vi "run.vi"(8 "error in (no error)":errorcluster, 11 "DL090409StageScaffold in":refnum<class "StageDL090409Scaffold.lvclass">) -> (0 "error out":errorcluster, 3 "DL090409StageScaffold out":refnum<class "StageDL090409Scaffold.lvclass">)   [LabVIEW 2010, in "StageDL090409Scaffold.lvclass"]
uses:
  StageDL090409Scaffold.lvclass
  main/labview_source/controls/undock_button.ctl
  internal_trigger_enum.ctl
  state_enum.ctl
  common/classes/SpaceVector/SpaceVector/SpaceVector.lvclass
  StageDL090409Scaffold.lvclass/StageDL090409Scaffold.ctl
  common/enumerations/top-level_component_type_enum.ctl
  GenericStage/GenericStage/trigger_enum.ctl
  GenericStage/GenericStage/translation_mode_enum.ctl
  stored_data_cluster.ctl
  common/classes/Image/Image/Image.lvclass
  Display/GenericDisplay/GenericDisplay/GenericDisplay.lvclass
  common/classes/GenericToplevelComponent/GenericToplevelComponent/trigger_type_enum.ctl
  GenericStage/GenericStage/GenericStage.lvclass
  common/classes/GenericToplevelComponent/GenericToplevelComponent/GenericToplevelComponent.lvclass
  common/classes/ErrorController/ErrorController/class_data.vi
  common/classes/ErrorController/ErrorController/ErrorController.lvclass
panel:
  in  "button:undock":T1
  in  "Tab Control":enum32{"User", "Debug", "About"}(tab)
  out "current x":dbl[unit] caption="x"
  out "current y":dbl[unit] caption="y"
  out "current z":dbl[unit] caption="z"
  in  "setOriginButton":bool
  in  "step x":dbl[unit] caption="x"
  in  "step y":dbl[unit] caption="y"
  in  "step z":dbl[unit] caption="z"
  in  "stepButton":bool
  in  "returnToOriginButton":bool
  in  "Stored positions":i32(listbox)
  in  "Description":string
  in  "store button":bool
  out "position image":T2(plugin-control)
  in  "go to stored button":bool
  in  "remove stored item":bool
  out "finished?":bool
  out "last trigger":T3=enum."initialise"
  out "state":T4
  out "statemachine loop counter":i32
  out "event loop error":errorcluster
  out "statemachine error":errorcluster
  out "event loop counter":i32
  # "Move"
  # "Current position"
  # "StageDL090409Scaffold (or child class)\n\nimplemented by: Dominik Langer, University of Zurich\nmodified by: Marcel van 't Hoff, University of Zurich"
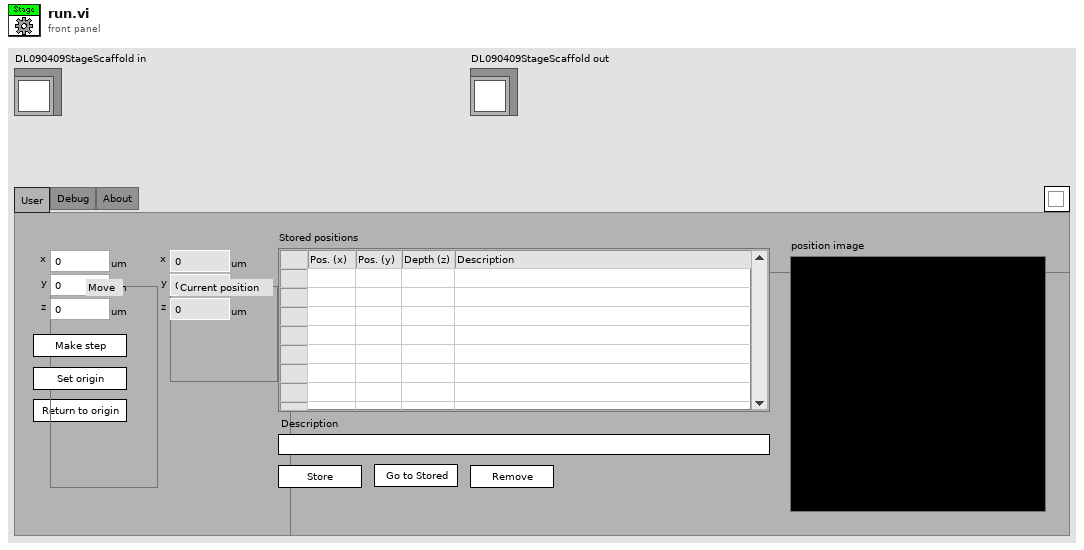
[diagram p1: front panel]
types:
  T1 = typedef "undock_button.ctl" = bool
  T2 = typedef "IMAQ Image.ctl" = refnum<image>
  T3 = typedef "StageDL090409Scaffold.lvclass/internal_trigger_enum.ctl" = enum16{"NULL", "initialise", "terminate", "move", "update position", "set origin", "return to origin", "attach observer", "detach observer", "go to stored"}
  T4 = typedef "StageDL090409Scaffold.lvclass/state_enum.ctl" = enum16{"idle", "moving"}
  T5 = typedef "top-level_component_type_enum.ctl" = enum16{"undefined", "ImagingMode", "ScanHead", "DAQ", "ImageAssembler", "Display", "DataCollection", "Analyser", "Stimulator", "ExperimentController", "Instrument", "Stage"}
  T6 = typedef "GenericStage.lvclass/trigger_enum.ctl" = enum16{"NULL", "move", "update position", "set origin", "return to origin"}
  T7 = typedef "GenericStage.lvclass/translation_mode_enum.ctl" = enum16{"DON'T MOVE", "relative", "absolute"}
  T8 = typedef "StageDL090409Scaffold.lvclass/stored_data_cluster.ctl" = cluster{"stored position":refnum<class "SpaceVector.lvclass">, "description":string, "position image":refnum<class "Image.lvclass">}
  T9 = typedef "trigger_type_enum.ctl" = enum8{"external", "internal", "common"}
  T10 = typedef "main_trigger_enum.ctl" = enum16{"NULL", "initialise", "terminate", "start", "stop", "change objective", "change experimentController", "change imagingMode", "save notebook", "started saving", "finished saving", "expCtr ready", "expCtr missing", "imgMd ready", "imgMd missing", "scanHd ready", "scanHd missing", "DAQ ready", "DAQ missing", "imgAsm ready", "imgAsm missing", "dataColl ready", "dataColl missing", "display ready", "display missing", "analysr ready", "analysr missing", "instrmnt ready", "instrmnt missing", "stimltr ready", "stimltr missing", "stage ready", "stage missing"}
  T11 = typedef "GenericToplevelComponent.lvclass/common_trigger_enum.ctl" = enum16{"NULL", "initialise", "terminate", "fetch command", "fetch data", "attach observer", "register as observer", "detach observer", "acknowledge", "start", "stop", "sweep started", "sweep finished", "experiment started", "experiment stopped"}
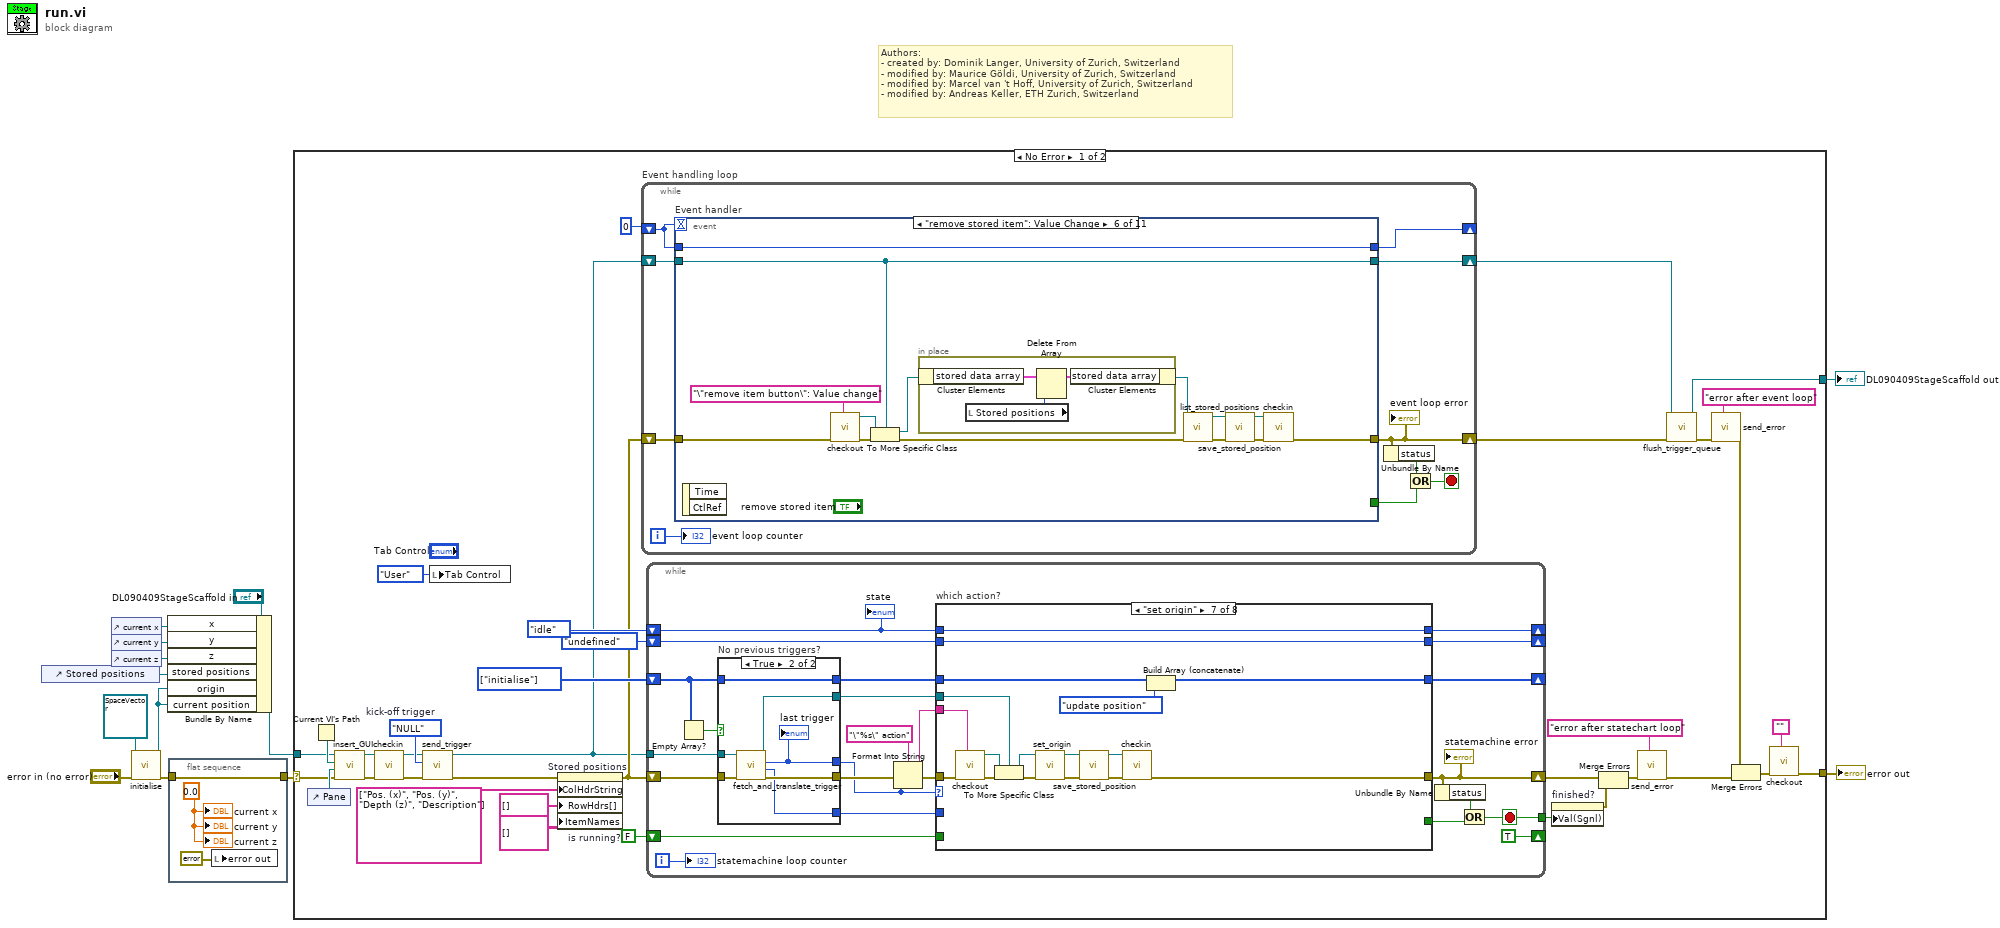
[diagram p0: block diagram]
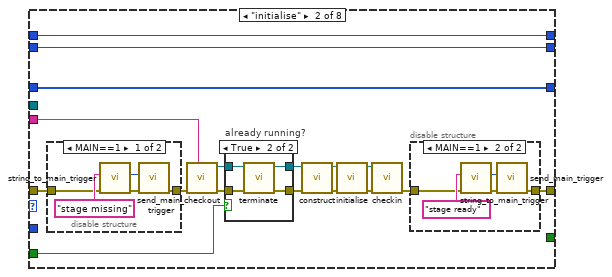
[diagram p3: hidden frame]
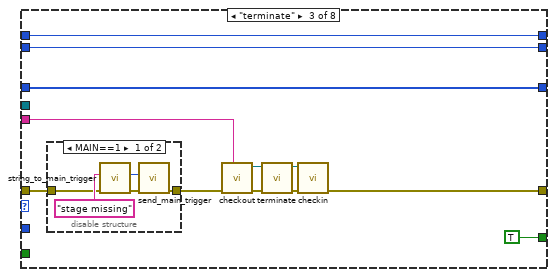
[diagram p7: hidden frame]
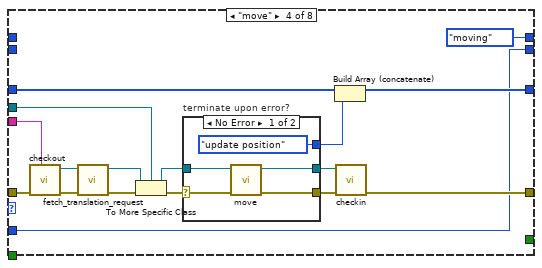
[diagram p9: hidden frame]
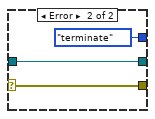
[diagram p10: hidden frame]
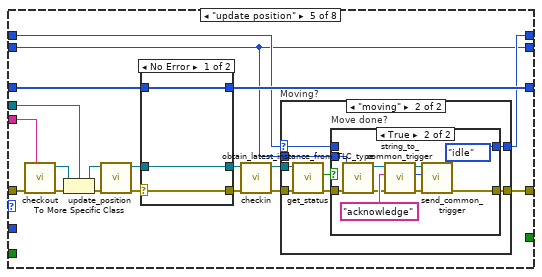
[diagram p11: hidden frame]
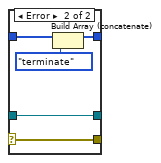
[diagram p14: hidden frame]
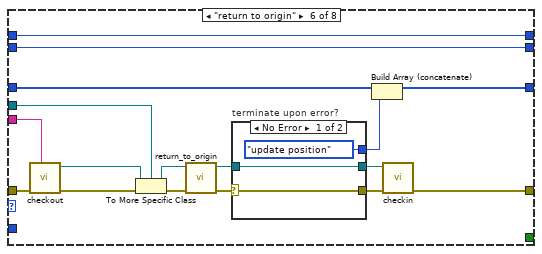
[diagram p15: hidden frame]
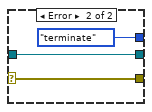
[diagram p16: hidden frame]
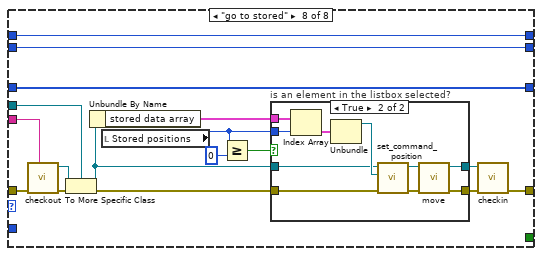
[diagram p17: hidden frame]
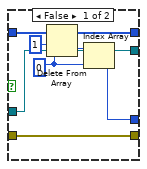
[diagram p19: hidden frame]
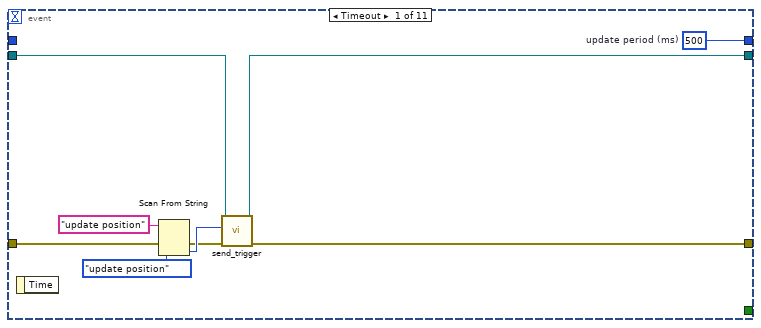
[diagram p20: hidden frame]
diagram:
  # "Authors: \n- created by: Dominik Langer, University of Zurich, Switzerland\n- modified by: Maurice Göldi, University of Zurich, Switzerland\n- modified by: Marcel van 't Hoff, University of Zurich, Switzerland\n- modified by: Andreas Keller, ETH Zurich, Switzerland"
  n1 = control-ref of="Stored positions"() -> (w6:refnum<vi>)
  n2 = control-ref of="current x"() -> (w9:refnum<vi>)
  n3 = control-ref of="current y"() -> (w8:refnum<vi>)
  n4 = control-ref of="current z"() -> (w7:refnum<vi>)
  n5 = call "initialise.vi"("error in (no error)"="error in (no error)", "SpaceVector in"=refnum<class "SpaceVector.lvclass"> refnum ("current position")) -> ("error out"=w2:errorcluster, "SpaceVector out"=w4:refnum<class "SpaceVector.lvclass">)  [unwired: 3 in, 5 out]
  n6 = Bundle By Name(cluster="DL090409StageScaffold in", "x"=w9, "y"=w8, "z"=w7, "stored positions"=w6, "origin"=w4, "current position"=w4) -> (w10:refnum<class "StageDL090409Scaffold.lvclass">)
  n7 = flat-sequence {
    tunnel: w2 -> [w15]
    tunnel: [w15] -> w1
    frame #0 {
      w16 = dbl[unit] 0.0 ("current x")
      n8 = local write "error out"(errorcluster {"status"=FALSE, "code"=0, "source"=""} ("error in (no error)")) -> ()
      "current x" <- w16
      "current y" <- w16
      "current z" <- w16
    }
  }
  n9 = case shown="No Error" w1 {
    selector: w1 -> [w44 w458]
    tunnel: [w50 w458] -> w13
    tunnel: [w31 w457] -> w12
    tunnel: w10 -> [w47 w457]
    frame No Error {
      w29 = FALSE  # is running?
      w30 = T3[] [enum."initialise"] items=["NULL", "initialise", "terminate", "move", "update position", "set origin", "return to origin", "attach observer", "detach observer", "go to stored"]
      w40 = trigger_enum."NULL"  # kick-off trigger
      n10 = control-ref of="Pane"() -> (w46:refnum<vi>)
      n11 = Current VI's Path() -> (path=w48:path)
      n12 = call-dynamic "insert_GUI.vi"("error in (no error)"=w44, "Pane"=w46, "VI path"=w48, "GenericComponent in"=w47) -> ("error out"=w22:errorcluster, "GenericComponent out"=w21:refnum<class "StageDL090409Scaffold.lvclass">)  [unwired: 6 in]
      n13 = call-dynamic "checkin.vi"("error in (no error)"=w22, "GenericStage in"=w21) -> ("error out"=w38:errorcluster, "GenericStage out"=w37:refnum<class "StageDL090409Scaffold.lvclass">)  [unwired: 8 in]
      n14 = call-dynamic "send_trigger.vi"("error in (no error)"=w38, "trigger"=w40, "GenericStage in"=w37) -> ("error out"=w41:errorcluster, "GenericStage out"=w19:refnum<class "StageDL090409Scaffold.lvclass">)  [unwired: 7 in]
      n15 = local write "Tab Control"(enum32{"User", "Debug", "About"}."User" ("Tab Control")) -> ()
      n16 = property on="Stored positions" class="MCListbox (strict)"(error in=w41, "ColHdrString"=string[] ["Pos. (x)", "Pos. (y)", "Depth (z)", "Description"] ("Row Header Strings[]"), "RowHdrs[]"=string[] [] ("Row Header Strings[]"), "ItemNames"=string[][] [] ("Item Names")) -> (error out=w20:errorcluster)  [unwired: 1 in, 1 out]
      n17 = while "Event handling loop" {
        shift-right: [w300] -> _
        shift-left: 0 -> [w301]
        shift-right: [w296] -> w33
        shift-left: w20 -> [w299]
        shift-right: [w297] -> w34
        shift-left: w19 -> [w298]
        i -> [w292]
        stop <- w293 stop-if-true
        n18 = event "Event handler" shown="[5] \"remove stored item\": Value Change" {
          selector: _ -> [_ _ _ _ _ _ _ _ _ _ _]
          dyn-events: _ -> [_ _ _ _ _ _ _ _ _ _ _]
          timeout: w301 -> [_ _ _ _ _ _ _ _ _ _ _]
          tunnel: w301 -> [_ w319 w331 w340 w372 w399 w413 w428 w435 w452 w456]
          tunnel: [w310 w319 w331 w340 w372 w399 w413 w428 w435 w452 w456] -> w300
          tunnel: w299 -> [w303 w317 w330 w334 w371 w394 w412 w421 w434 w451 w455]
          tunnel: [w307 w311 w324 w337 w347 w393 w409 w415 w433 w447 w455] -> w296
          tunnel: [_ _ _ _ _ _ _ _ _ _ TRUE] -> w294
          tunnel: w298 -> [w309 w318 w323 w339 w368 w398 w408 w417 w432 w444 w453]
          tunnel: [w308 w312 w321 w338 w368 w398 w407 w417 w431 w443 w453] -> w297
          event Timeout {
            w310 = 500  # update period (ms)
            n19 = event-data() -> ()  [unwired: 2 out]
            n20 = Scan From String(input string="update position", error in=w303, default 1=trigger_enum."update position" ("trigger")) -> (error out=w302:errorcluster, output 1=w304:T6)  [unwired: 2 in, 2 out]
            n21 = call-dynamic "send_trigger.vi"("error in (no error)"=w302, "trigger"=w304, "GenericStage in"=w309) -> ("error out"=w307:errorcluster, "GenericStage out"=w308:refnum<class "StageDL090409Scaffold.lvclass">)  [unwired: 7 in]
          }
          event "setOriginButton": Value Change {
            n22 = event-data() -> ()  [unwired: 3 out]
            n23 = Scan From String(input string="set origin", error in=w317, default 1=trigger_enum."set origin" ("trigger")) -> (error out=w316:errorcluster, output 1=w313:T6)  [unwired: 2 in, 2 out]
            n24 = call-dynamic "send_trigger.vi"("error in (no error)"=w316, "trigger"=w313, "GenericStage in"=w318) -> ("error out"=w311:errorcluster, "GenericStage out"=w312:refnum<class "StageDL090409Scaffold.lvclass">)  [unwired: 7 in]
          }
          event "stepButton": Value Change {
            n25 = event-data() -> ()  [unwired: 3 out]
            n26 = call "initialise.vi"("z"="step z", "error in (no error)"=w330, "y"="step y", "x"="step x", "SpaceVector in"=refnum<class "SpaceVector.lvclass"> refnum ("current position")) -> ("error out"=w325:errorcluster, "SpaceVector out"=w326:refnum<class "SpaceVector.lvclass">)  [unwired: 5 in]
            n27 = call-dynamic "send_translation_request.vi"("error in (no error)"=w325, "translation mode"=translation_mode_enum."relative", "translation vector"=w326, "GenericStage in"=w323) -> ("error out"=w324:errorcluster, "GenericStage out"=w321:refnum<class "StageDL090409Scaffold.lvclass">)  [unwired: 6 in]
          }
          event "returnToOriginButton": Value Change {
            n28 = event-data() -> ()  [unwired: 3 out]
            n29 = Scan From String(input string="return to origin", error in=w334, default 1=trigger_enum."return to origin" ("trigger")) -> (error out=w333:errorcluster, output 1=w332:T6)  [unwired: 2 in, 2 out]
            n30 = call-dynamic "send_trigger.vi"("error in (no error)"=w333, "trigger"=w332, "GenericStage in"=w339) -> ("error out"=w337:errorcluster, "GenericStage out"=w338:refnum<class "StageDL090409Scaffold.lvclass">)  [unwired: 7 in]
          }
          event "store button": Value Change {
            n31 = event-data() -> ()  [unwired: 3 out]
            n32 = call "checkout.vi"("locked by?"="\"store button\": Value change", "error in (no error)"=w371) -> ("error out"=w370:errorcluster, "GenericStage out"=w369:refnum<class "GenericStage.lvclass">)  [unwired: 8 in]
            n33 = To More Specific Class(target class=w368, reference=w369, error in=w370) -> (specific class reference=w355:refnum<class "StageDL090409Scaffold.lvclass">, error out=w363:errorcluster)
            n34 = Unbundle By Name(w355) -> ("stored data array"=w357:T8[], "current position"=w360:refnum<class "SpaceVector.lvclass">)
            n35 = call "create.vi"("error in (no error)"=w363) -> ("error out"=w362:errorcluster, "Image out"=w361:refnum<class "Image.lvclass">)  [unwired: 9 in]
            n36 = disable-structure shown="DISPLAY==1" {
              disable-tunnel: w362 -> [w375 w378]
              disable-tunnel: [w374 w378] -> w352
              disable-tunnel: [w373 _] -> w350
              frame condition #0 (active) {
                n37 = call "obtain_latest_instance.vi"("error in (no error)"=w375) -> ("error out"=w377:errorcluster, "GenericDisplay out"=w376:refnum<class "GenericDisplay.lvclass">)  [unwired: 9 in]
                n38 = call-dynamic "get_current_RGB_image.vi"("error in (no error)"=w377, "GenericDisplay in"=w376) -> ("error out"=w374:errorcluster, "RGB image"=w373:refnum<class "Image.lvclass">)  [unwired: 7 in, 1 out]
              }
              frame condition #1 {
              }
            }
            n39 = call-dynamic "is_empty.vi"("error in (no error)"=w352, "Image in"=w350) -> ("error out"=w351:errorcluster, "emtpy?"=w348:bool, "Image out"=w349:refnum<class "Image.lvclass">)  [unwired: 7 in]
            n40 = case shown="False" w348 {
              tunnel: [w383 w385] -> w367
              tunnel: [w382 w384] -> w365
              tunnel: w361 -> [w381 w384]
              tunnel: w351 -> [w380 w385]
              tunnel: w349 -> [w379 _]
              frame False {
                n41 = call "copy.vi"("error in (no error)"=w380, "image to copy (source)"=w379, "Image in (target)"=w381) -> ("error out"=w383:errorcluster, "Image out"=w382:refnum<class "Image.lvclass">)  [unwired: 7 in]
              }
              frame True {
              }
            }
            n42 = call-dynamic "get_IMAQ_ref.vi"("error in (no error)"=w367, "Image.lvclass in"=w365) -> ("error out"=w346:errorcluster, "Image"=→"position image":T2, "Image.lvclass out"=w358:refnum<class "Image.lvclass">)  [unwired: 5 in, 2 out]
            n43 = Bundle(cluster=T8 {"stored position"=refnum, "description"="", "position image"=refnum} ("stored data"), "stored position"=w360, "description"="Description", "position image"=w358) -> (w356:T8)
            n44 = Build Array (concatenate)(w357, w356) -> (w353:T8[])
            n45 = Bundle By Name(cluster=w355, "stored data array"=w353) -> (w345:refnum<class "StageDL090409Scaffold.lvclass">)
            n46 = call-dynamic "list_stored_positions.vi"("error in (no error)"=w346, "StageDL090409Scaffold in"=w345) -> ("error out"=w344:errorcluster, "StageDL090409Scaffold out"=w343:refnum<class "StageDL090409Scaffold.lvclass">)  [unwired: 8 in]
            n47 = call-dynamic "save_stored_position.vi"("error in (no error)"=w344, "StageDL090409Scaffold in"=w343) -> ("error out"=w341:errorcluster, "StageDL090409Scaffold out"=w342:refnum<class "StageDL090409Scaffold.lvclass">)  [unwired: 8 in]
            n48 = call-dynamic "checkin.vi"("error in (no error)"=w341, "GenericStage in"=w342) -> ("error out"=w347:errorcluster)  [unwired: 8 in, 1 out]
          }
          event "remove stored item": Value Change {
            n49 = event-data() -> ()  [unwired: 3 out]
            n50 = call "checkout.vi"("locked by?"="\"remove item button\": Value change", "error in (no error)"=w394) -> ("error out"=w397:errorcluster, "GenericStage out"=w395:refnum<class "GenericStage.lvclass">)  [unwired: 8 in]
            n51 = To More Specific Class(target class=w398, reference=w395, error in=w397) -> (specific class reference=w391:refnum<class "StageDL090409Scaffold.lvclass">, error out=w392:errorcluster)
            n52 = in-place {
              n53 = in-place-cluster #1(w391) -> ("stored data array"=w401:T8[])
              n54 = local read "Stored positions"() -> (w402:i32)
              n55 = Delete From Array(array=w401, index=w402) -> (array with subset deleted=w400:T8[])  [unwired: 1 in, 1 out]
              n56 = in-place-cluster #1("stored data array"=w400) -> (w390:refnum<class "StageDL090409Scaffold.lvclass">)
            }
            n57 = call-dynamic "list_stored_positions.vi"("error in (no error)"=w392, "StageDL090409Scaffold in"=w390) -> ("error out"=w389:errorcluster, "StageDL090409Scaffold out"=w387:refnum<class "StageDL090409Scaffold.lvclass">)  [unwired: 8 in]
            n58 = call-dynamic "save_stored_position.vi"("error in (no error)"=w389, "StageDL090409Scaffold in"=w387) -> ("error out"=w388:errorcluster, "StageDL090409Scaffold out"=w386:refnum<class "StageDL090409Scaffold.lvclass">)  [unwired: 8 in]
            n59 = call-dynamic "checkin.vi"("error in (no error)"=w388, "GenericStage in"=w386) -> ("error out"=w393:errorcluster)  [unwired: 8 in, 1 out]
          }
          event "go to stored button": Value Change {
            n60 = event-data() -> ()  [unwired: 2 out]
            n61 = Scan From String(input string="go to stored", error in=w412, default 1=internal_trigger_enum."update position" ("internal trigger")) -> (error out=w410:errorcluster, output 1=w406:T3)  [unwired: 2 in, 2 out]
            n62 = To Variant(anything=w406) -> (Variant=w405:variant)
            n63 = call-dynamic "send_generic_trigger.vi"("error in (no error)"=w410, "trigger type"=trigger_type_enum."internal", "trigger variant"=w405, "GenericToplevelComponent in"=w408) -> ("error out"=w409:errorcluster, "GenericToplevelComponent out"=w407:refnum<class "StageDL090409Scaffold.lvclass">)  [unwired: 4 in, 2 out]
          }
          event "Stored positions": Mouse Up {
            n64 = event-data() -> ()  [unwired: 2 out]
            n65 = call "checkout.vi"("locked by?"="stored positions: Mouse Down", "error in (no error)"=w421) -> ("error out"=w422:errorcluster, "GenericStage out"=w418:refnum<class "GenericStage.lvclass">)  [unwired: 8 in]
            n66 = To More Specific Class(target class=w417, reference=w418, error in=w422) -> (specific class reference=w414:refnum<class "StageDL090409Scaffold.lvclass">, error out=w420:errorcluster)
            n67 = Unbundle By Name(w414) -> ("stored data array"=w427:T8[])
            n68 = Index Array(array=w427, index="Stored positions") -> (element=w426:T8)
            n69 = Unbundle By Name(w426) -> ("position image"=w425:refnum<class "Image.lvclass">)
            n70 = call-dynamic "get_IMAQ_ref.vi"("error in (no error)"=w420, "Image.lvclass in"=w425) -> ("error out"=w416:errorcluster, "Image"=w424:T2)  [unwired: 5 in, 3 out]
            n71 = local write "position image"(w424) -> ()
            n72 = call-dynamic "checkin.vi"("error in (no error)"=w416, "GenericStage in"=w414) -> ("error out"=w415:errorcluster)  [unwired: 8 in, 1 out]
          }
          event Value Change {
            n73 = event-data() -> ()  [unwired: 2 out]
            n74 = Current VI's Path() -> (path=w429:path)
            n75 = call-dynamic "undock.vi"("error in (no error)"=w434, "undock?"="button:undock", "VI path"=w429, "GenericComponent in"=w432) -> ("error out"=w433:errorcluster, "GenericComponent out"=w431:refnum<class "StageDL090409Scaffold.lvclass">)  [unwired: 6 in]
          }
          event "Stored positions": Edit Cell {
            n76 = event-data() -> ("Coords.Row"=w440:i32, "Coords.Column"=w442:i32, "String"=w441:string)  [unwired: 1 out]
            n77 = call "checkout.vi"("locked by?"="Stored position edited: Value Change", "error in (no error)"=w451) -> ("error out"=w448:errorcluster, "GenericStage out"=w449:refnum<class "GenericStage.lvclass">)  [unwired: 8 in]
            n78 = To More Specific Class(target class=w444, reference=w449, error in=w448) -> (specific class reference=w446:refnum<class "StageDL090409Scaffold.lvclass">, error out=w445:errorcluster)
            n79 = call-dynamic "change_stored_position.vi"("Row"=w440, "String"=w441, "Column"=w442, "error in (no error)"=w445, "specific class reference"=w446, "StageDL090409Scaffold in"=w444) -> ("error out"=w439:errorcluster, "specific class reference out"=w436:refnum<class "StageDL090409Scaffold.lvclass">, "StageDL090409Scaffold out"=w443:refnum<class "StageDL090409Scaffold.lvclass">)  [unwired: 3 in]
            n80 = call-dynamic "save_stored_position.vi"("error in (no error)"=w439, "StageDL090409Scaffold in"=w436) -> ("error out"=w437:errorcluster, "StageDL090409Scaffold out"=w438:refnum<class "StageDL090409Scaffold.lvclass">)  [unwired: 8 in]
            n81 = call-dynamic "checkin.vi"("error in (no error)"=w437, "GenericStage in"=w438) -> ("error out"=w447:errorcluster)  [unwired: 8 in, 1 out]
          }
          event "finished?": Value Change {
            n82 = event-data() -> ()  [unwired: 3 out]
          }
        }
        "event loop error" <- w296
        n83 = Unbundle By Name(w296) -> ("status"=w295:bool)
        n84 = Or(x=w295, y=w294) -> (x .or. y?=w293:bool)
        "event loop counter" <- w292
      }
      n85 = while {
        shift-right: [w61] -> w25
        shift-left: w20 -> [w76]
        shift-right: [w67] -> _
        shift-left: w30 -> [w73]
        shift-right: [TRUE ("is running?")] -> _
        shift-left: w29 -> [w64]
        tunnel: w19 -> [w75]
        tunnel: [w58] -> w28
        shift-right: [w56] -> _
        shift-left: state_enum."idle" ("state") -> [w57]
        shift-right: [w54] -> _
        shift-left: top-level_component_type_enum."undefined" ("sender TLC type") -> [w53]
        i -> [w55]
        stop <- w58 stop-if-true
        n86 = Empty Array?(array=w73) -> (empty?=w74:bool)
        n87 = case "No previous triggers?" shown="True" w74 {
          tunnel: w75 -> [w284 w288]
          tunnel: w76 -> [w282 w290]
          tunnel: [w284 w287] -> w68
          tunnel: [w280 w285] -> w70
          tunnel: [_ w286] -> w62
          tunnel: [w282 w289] -> w71
          tunnel: w73 -> [w283 w291]
          tunnel: [w279 w291] -> w66
          frame False {
            w277 = 0 ("index")
            n88 = Delete From Array(array=w283, length=1, index=w277) -> (deleted portion=w281:T3[], array with subset deleted=w279:T3[])
            n89 = Index Array(array=w281, index=w277) -> (element=w280:T3)
          }
          frame True {
            n90 = call-dynamic "fetch_and_translate_trigger.vi"("error in (no error)"=w290, "StageDL090409Scaffold in"=w288) -> ("error out"=w289:errorcluster, "sender TLC type"=w286:T5, "statechart trigger"=w285:T3, "StageDL090409Scaffold out"=w287:refnum<class "StageDL090409Scaffold.lvclass">)  [unwired: 6 in]
            "last trigger" <- w285
          }
        }
        n91 = Format Into String(format string="\"%s\" action", error in=w71, w70) -> (resulting string=w65:string, error out=w69:errorcluster)  [unwired: 1 in]
        n92 = case "which action?" shown="\"set origin\"" w70 {
          tunnel: [w79 w86 w124 w141 w165 w219 w241 w250] -> w61
          tunnel: w69 -> [w79 w84 w117 w148 w176 w223 w245 w251]
          tunnel: w68 -> [_ _ _ w145 w175 w222 w242 w249]
          tunnel: [w80 w85 w127 w139 w169 w211 w239 w264] -> w67
          tunnel: w66 -> [w80 w85 w127 w140 w170 w210 w240 w264]
          tunnel: w65 -> [_ w91 w121 w149 w177 w224 w237 w248]
          tunnel: w64 -> [_ w92 _ _ _ _ _ _]
          tunnel: w62 -> [_ _ _ w134 _ _ _ _]
          tunnel: [_ _ TRUE _ _ _ _ _] -> w60
          tunnel: [w78 w82 w119 state_enum."moving" ("state") w164 w209 w236 w263] -> w56
          tunnel: w57 -> [w78 w82 w119 _ w161 w209 w236 w263]
          tunnel: [w77 w81 w118 w134 w159 w208 w235 w262] -> w54
          tunnel: w53 -> [w77 w81 w118 _ w159 w208 w235 w262]
          frame "NULL", Default {
          }
          frame "initialise" {
            n93 = disable-structure shown="MAIN==1" {
              disable-tunnel: w84 -> [w99 w103]
              disable-tunnel: [w102 w103] -> w83
              frame condition #0 (active) {
                n94 = call "string_to_main_trigger.vi"("error in (no error)"=w99, "trigger string"="stage missing") -> ("error out"=w100:errorcluster, "main trigger"=w98:T10)  [unwired: 8 in]
                n95 = call "send_main_trigger.vi"("error in (no error)"=w100, "trigger"=w98) -> ("error out"=w102:errorcluster)  [unwired: 9 in]
              }
              frame condition #1 {
              }
            }
            n96 = call "checkout.vi"("locked by?"=w91, "error in (no error)"=w83) -> ("error out"=w93:errorcluster, "GenericStage out"=w90:refnum<class "GenericStage.lvclass">)  [unwired: 8 out]
            n97 = case "already running?" shown="True" w92 {
              tunnel: w93 -> [w110 w114]
              tunnel: w90 -> [w111 w115]
              tunnel: [w110 w113] -> w88
              tunnel: [w111 w112] -> w89
              frame False {
              }
              frame True {
                n98 = call-dynamic "terminate.vi"("error in (no error)"=w114, "GenericPlugin in"=w115) -> ("error out"=w113:errorcluster, "GenericPlugin out"=w112:refnum<class "GenericStage.lvclass">)  [unwired: 8 out]
              }
            }
            n99 = call-dynamic "construct.vi"("error in (no error)"=w88, "GenericPlugin in"=w89) -> ("error out"=w95:errorcluster, "GenericPlugin out"=w94:refnum<class "GenericStage.lvclass">)  [unwired: 2 in, 6 out]
            n100 = call-dynamic "initialise.vi"("error in (no error)"=w95, "GenericPlugin in"=w94) -> ("error out"=w96:errorcluster, "GenericPlugin out"=w97:refnum<class "GenericStage.lvclass">)  [unwired: 8 out]
            n101 = call-dynamic "checkin.vi"("error in (no error)"=w96, "GenericStage in"=w97) -> ("error out"=w87:errorcluster)  [unwired: 8 in, 1 out]
            n102 = disable-structure shown="MAIN==1" {
              disable-tunnel: [w104 w109] -> w86
              disable-tunnel: w87 -> [w104 w107]
              frame condition #0 {
              }
              frame condition #1 (active) {
                n103 = call "string_to_main_trigger.vi"("error in (no error)"=w107, "trigger string"="stage ready") -> ("error out"=w106:errorcluster, "main trigger"=w105:T10)  [unwired: 8 in]
                n104 = call "send_main_trigger.vi"("error in (no error)"=w106, "trigger"=w105) -> ("error out"=w109:errorcluster)  [unwired: 9 in]
              }
            }
          }
          frame "terminate" {
            n105 = disable-structure shown="MAIN==1" {
              disable-tunnel: w117 -> [w129 w133]
              disable-tunnel: [w132 w133] -> w116
              frame condition #0 (active) {
                n106 = call "string_to_main_trigger.vi"("error in (no error)"=w129, "trigger string"="stage missing") -> ("error out"=w130:errorcluster, "main trigger"=w128:T10)  [unwired: 8 in]
                n107 = call "send_main_trigger.vi"("error in (no error)"=w130, "trigger"=w128) -> ("error out"=w132:errorcluster)  [unwired: 9 in]
              }
              frame condition #1 {
              }
            }
            n108 = call "checkout.vi"("locked by?"=w121, "error in (no error)"=w116) -> ("error out"=w125:errorcluster, "GenericStage out"=w123:refnum<class "GenericStage.lvclass">)  [unwired: 8 out]
            n109 = call-dynamic "terminate.vi"("error in (no error)"=w125, "GenericPlugin in"=w123) -> ("error out"=w126:errorcluster, "GenericPlugin out"=w122:refnum<class "GenericStage.lvclass">)  [unwired: 8 out]
            n110 = call-dynamic "checkin.vi"("error in (no error)"=w126, "GenericStage in"=w122) -> ("error out"=w124:errorcluster)  [unwired: 8 in, 1 out]
          }
          frame "move" {
            n111 = call "checkout.vi"("locked by?"=w149, "error in (no error)"=w148) -> ("error out"=w150:errorcluster, "GenericStage out"=w147:refnum<class "GenericStage.lvclass">)  [unwired: 8 out]
            n112 = call-dynamic "fetch_translation_request.vi"("error in (no error)"=w150, "GenericStage in"=w147) -> ("error out"=w146:errorcluster, "GenericStage out"=w144:refnum<class "GenericStage.lvclass">)  [unwired: 8 out]
            n113 = To More Specific Class(target class=w145, reference=w144, error in=w146) -> (specific class reference=w137:refnum<class "StageDL090409Scaffold.lvclass">, error out=w136:errorcluster)
            n114 = case "terminate upon error?" shown="No Error" w136 {
              selector: w136 -> [w154 w158]
              tunnel: w137 -> [w155 w157]
              tunnel: [w153 w157] -> w143
              tunnel: [w152 w158] -> w142
              tunnel: [internal_trigger_enum."update position" ("internal trigger enum") internal_trigger_enum."terminate" ("internal trigger enum")] -> w138
              frame No Error {
                n115 = call-dynamic "move.vi"("error in (no error)"=w154, "DL090409StageScaffold in"=w155) -> ("error out"=w152:errorcluster, "DL090409StageScaffold out"=w153:refnum<class "StageDL090409Scaffold.lvclass">)  [unwired: 8 out]
              }
              frame Error {
              }
            }
            n116 = Build Array (concatenate)(w140, w138) -> (w139:T3[])
            n117 = call-dynamic "checkin.vi"("error in (no error)"=w142, "GenericStage in"=w143) -> ("error out"=w141:errorcluster)  [unwired: 8 in, 1 out]
          }
          frame "update position" {
            n118 = call "checkout.vi"("locked by?"=w177, "error in (no error)"=w176) -> ("error out"=w167:errorcluster, "GenericStage out"=w168:refnum<class "GenericStage.lvclass">)  [unwired: 8 out]
            n119 = To More Specific Class(target class=w175, reference=w168, error in=w167) -> (specific class reference=w174:refnum<class "StageDL090409Scaffold.lvclass">, error out=w173:errorcluster)
            n120 = call-dynamic "update_position.vi"("error in (no error)"=w173, "DL090409StageScaffold in"=w174) -> ("error out"=w171:errorcluster, "DL090409StageScaffold out"=w172:refnum<class "StageDL090409Scaffold.lvclass">)  [unwired: 8 out]
            n121 = case shown="No Error" w171 {
              selector: w171 -> [w200 w207]
              tunnel: w172 -> [w201 w206]
              tunnel: [w201 w206] -> w163
              tunnel: [w200 w207] -> w162
              tunnel: w170 -> [w202 w205]
              tunnel: [w202 w204] -> w169
              frame No Error {
              }
              frame Error {
                n122 = Build Array (concatenate)(w205, internal_trigger_enum."terminate" ("internal trigger enum")) -> (w204:T3[])
              }
            }
            n123 = call-dynamic "checkin.vi"("error in (no error)"=w162, "GenericStage in"=w163) -> ("error out"=w166:errorcluster, "GenericStage out"=w160:refnum<class "StageDL090409Scaffold.lvclass">)  [unwired: 8 in]
            n124 = case "Moving?" shown="\"moving\"" w161 {
              selector: w161 -> [w178 w181]
              tunnel: w166 -> [w179 w185]
              tunnel: [w179 w187] -> w165
              tunnel: [w178 w180] -> w164
              tunnel: w160 -> [_ w186]
              tunnel: w159 -> [_ w183]
              frame "idle", Default {
              }
              frame "moving" {
                n125 = call-dynamic "get_status.vi"("error in (no error)"=w185, "StageDL090409Scaffold in"=w186) -> ("error out"=w184:errorcluster, "is happy?"=w182:bool)  [unwired: 7 in, 1 out]
                n126 = case "Move done?" shown="True" w182 {
                  tunnel: [w188 w199] -> w187
                  tunnel: w184 -> [w188 w198]
                  tunnel: w183 -> [_ w197]
                  tunnel: w181 -> [w189 _]
                  tunnel: [w189 state_enum."idle" ("state")] -> w180
                  frame False {
                  }
                  frame True {
                    n127 = call "obtain_latest_instance_from_TLC_type.vi"("error in (no error)"=w198, "top-level component type"=w197) -> ("error out"=w194:errorcluster, "GenericToplevelComponent.lvclass"=w190:refnum<class "GenericToplevelComponent.lvclass">)  [unwired: 8 in]
                    n128 = call-dynamic "string_to_common_trigger.vi"("error in (no error)"=w194, "trigger string"="acknowledge", "GenericToplevelComponent in"=w190) -> ("error out"=w193:errorcluster, "trigger"=w191:T11, "GenericToplevelComponent out"=w192:refnum<class "GenericToplevelComponent.lvclass">)  [unwired: 6 in]
                    n129 = call-dynamic "send_common_trigger.vi"("error in (no error)"=w193, "trigger"=w191, "GenericToplevelComponent in"=w192) -> ("error out"=w199:errorcluster)  [unwired: 6 in, 2 out]
                  }
                }
              }
            }
          }
          frame "return to origin" {
            n130 = call "checkout.vi"("locked by?"=w224, "error in (no error)"=w223) -> ("error out"=w217:errorcluster, "GenericStage out"=w218:refnum<class "GenericStage.lvclass">)  [unwired: 8 out]
            n131 = To More Specific Class(target class=w222, reference=w218, error in=w217) -> (specific class reference=w216:refnum<class "StageDL090409Scaffold.lvclass">, error out=w215:errorcluster)
            n132 = call-dynamic "return_to_origin.vi"("error in (no error)"=w215, "StageDL090409Scaffold in"=w216) -> ("error out"=w214:errorcluster, "StageDL090409Scaffold out"=w213:refnum<class "StageDL090409Scaffold.lvclass">)  [unwired: 8 in]
            n133 = case "terminate upon error?" shown="No Error" w214 {
              selector: w214 -> [w226 w230]
              tunnel: w213 -> [w227 w229]
              tunnel: [w227 w229] -> w221
              tunnel: [w226 w230] -> w220
              tunnel: [internal_trigger_enum."update position" ("internal trigger enum") internal_trigger_enum."terminate" ("internal trigger enum")] -> w212
              frame No Error {
              }
              frame Error {
              }
            }
            n134 = Build Array (concatenate)(w210, w212) -> (w211:T3[])
            n135 = call-dynamic "checkin.vi"("error in (no error)"=w220, "GenericStage in"=w221) -> ("error out"=w219:errorcluster)  [unwired: 8 in, 1 out]
          }
          frame "set origin" {
            n136 = call "checkout.vi"("locked by?"=w237, "error in (no error)"=w245) -> ("error out"=w244:errorcluster, "GenericStage out"=w246:refnum<class "GenericStage.lvclass">)  [unwired: 8 out]
            n137 = To More Specific Class(target class=w242, reference=w246, error in=w244) -> (specific class reference=w247:refnum<class "StageDL090409Scaffold.lvclass">, error out=w243:errorcluster)
            n138 = call-dynamic "set_origin.vi"("error in (no error)"=w243, "StageDL090409Scaffold in"=w247) -> ("error out"=w234:errorcluster, "StageDL090409Scaffold out"=w232:refnum<class "StageDL090409Scaffold.lvclass">)  [unwired: 8 in]
            n139 = call-dynamic "save_stored_position.vi"("error in (no error)"=w234, "StageDL090409Scaffold in"=w232) -> ("error out"=w233:errorcluster, "StageDL090409Scaffold out"=w231:refnum<class "StageDL090409Scaffold.lvclass">)  [unwired: 8 in]
            n140 = call-dynamic "checkin.vi"("error in (no error)"=w233, "GenericStage in"=w231) -> ("error out"=w241:errorcluster)  [unwired: 8 in, 1 out]
            n141 = Build Array (concatenate)(w240, internal_trigger_enum."update position" ("internal trigger enum")) -> (w239:T3[])
          }
          frame "go to stored" {
            n142 = call "checkout.vi"("locked by?"=w248, "error in (no error)"=w251) -> ("error out"=w256:errorcluster, "GenericStage out"=w258:refnum<class "GenericStage.lvclass">)  [unwired: 8 in]
            n143 = To More Specific Class(target class=w249, reference=w258, error in=w256) -> (specific class reference=w260:refnum<class "StageDL090409Scaffold.lvclass">, error out=w257:errorcluster)
            n144 = Unbundle By Name(w260) -> ("stored data array"=w252:T8[])
            n145 = local read "Stored positions"() -> (w254:i32)
            n146 = Greater Or Equal?(x=w254, y=0) -> (x >= y?=w253:bool)
            n147 = case "is an element in the listbox selected?" shown="True" w253 {
              tunnel: w252 -> [_ w276]
              tunnel: [w266 w272] -> w259
              tunnel: w257 -> [w266 w270]
              tunnel: w254 -> [_ w269]
              tunnel: w260 -> [w265 w268]
              tunnel: [w265 w267] -> w261
              frame False {
              }
              frame True {
                n148 = Index Array(array=w276, index=w269) -> (element=w275:T8)
                n149 = Unbundle(w275) -> ("stored position"=w274:refnum<class "SpaceVector.lvclass">)  [unwired: 2 out]
                n150 = call-dynamic "set_command_position.vi"("error in (no error)"=w270, "command position"=w274, "DL090409StageScaffold.lvclass in"=w268) -> ("error out"=w273:errorcluster, "DL090409StageScaffold.lvclass out"=w271:refnum<class "StageDL090409Scaffold.lvclass">)  [unwired: 7 in]
                n151 = call-dynamic "move.vi"("error in (no error)"=w273, "DL090409StageScaffold in"=w271) -> ("error out"=w272:errorcluster, "DL090409StageScaffold out"=w267:refnum<class "StageDL090409Scaffold.lvclass">)  [unwired: 8 in]
              }
            }
            n152 = call-dynamic "checkin.vi"("error in (no error)"=w259, "GenericStage in"=w261) -> ("error out"=w250:errorcluster)  [unwired: 8 in, 1 out]
          }
        }
        "statemachine error" <- w61
        n153 = Unbundle By Name(w61) -> ("status"=w59:bool)
        n154 = Or(x=w59, y=w60) -> (x .or. y?=w58:bool)
        "state" <- w57
        "statemachine loop counter" <- w55
      }
      n155 = property on="finished?" class="Bool (strict)"("Val(Sgnl)"=w28) -> (error out=w24:errorcluster)  [unwired: 2 in, 1 out]
      n156 = Merge Errors(w25, w24) -> (w23:errorcluster)
      n157 = call "send_error.vi"("additional message"="error after statechart loop", "error in (no error)"=w23) -> ("error out"=w42:errorcluster)  [unwired: 9 in]
      n158 = call-dynamic "flush_trigger_queue.vi"("error in (no error)"=w33, "GenericToplevelComponent in"=w34) -> ("error out"=w32:errorcluster, "GenericToplevelComponent out"=w31:refnum<class "StageDL090409Scaffold.lvclass">)  [unwired: 8 in]
      n159 = call "send_error.vi"("additional message"="error after event loop", "error in (no error)"=w32) -> ("error out"=w43:errorcluster)  [unwired: 9 in]
      n160 = Merge Errors(w43, w42) -> (w51:errorcluster)
      n161 = call "checkout.vi"("locked by?"="", "error in (no error)"=w51) -> ("error out"=w50:errorcluster)  [unwired: 8 in, 1 out]
    }
    frame Error {
    }
  }
  "error out" <- w13
  "DL090409StageScaffold out" <- w12
